vi "globalTearDown.vi"(8 "error in (no error)":errorcluster, 11 "Single Core Complex Loopback in":refnum<class "Single Core Complex Loopback.lvclass">) -> (0 "error out":errorcluster, 3 "Single Core Complex Loopback out":refnum<class "Single Core Complex Loopback.lvclass">)   [LabVIEW 2020, in "Single Core Complex Loopback.lvclass"]
uses:
  Single Core Complex Loopback.lvclass
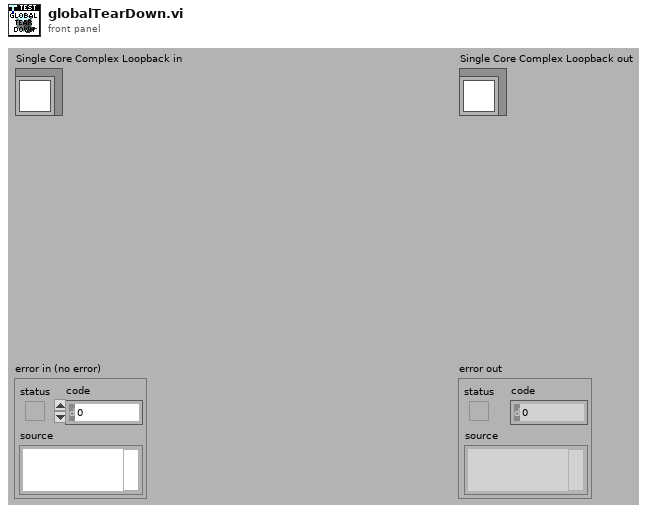
[diagram p1: front panel]
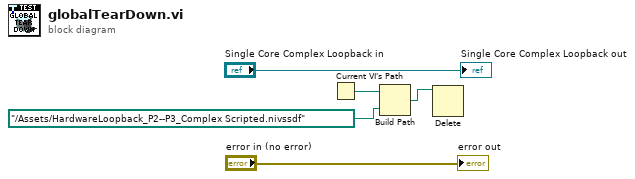
[diagram p0: block diagram]
diagram:
  n1 = Current VI's Path() -> (path=w3:path)
  n2 = Build Path(base path=w3, name or relative path=path "../Assets/HardwareLoopback_P2--P3_Complex Scripted.nivssdf" ("Hardware File Path")) -> (appended path=w1:path)
  n3 = Delete(path (use dialog)=w1) -> ()  [unwired: 4 in, 3 out]
  "error out" <- "error in (no error)"
  "Single Core Complex Loopback out" <- "Single Core Complex Loopback in"
